vi "1D数组排序[U32].vi"(8 "error in (no error)":errorcluster caption="错误输入（无错误）", 9 "升降序":enum16{"升序", "降序"}(ring), 11 "输入数组":u32[](array[numeric])) -> (0 "error out":errorcluster caption="错误输出", 2 "排序后索引":i32[](array[numeric]), 3 "排序后数组":u32[](array[numeric]))   [LabVIEW 2020]
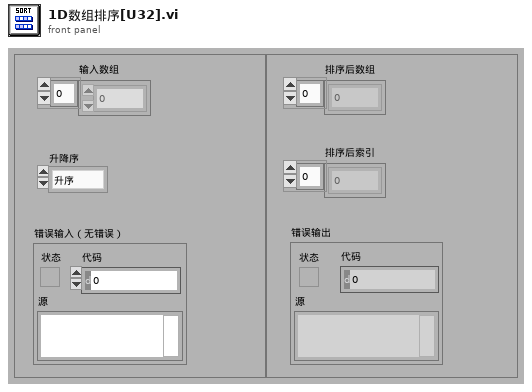
[diagram p1: front panel]
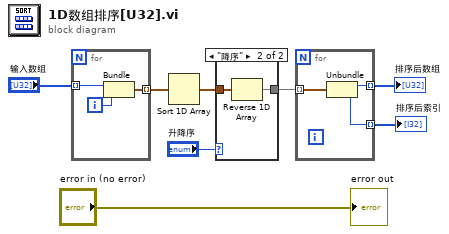
[diagram p0: block diagram]
diagram:
  n1 = for {
    tunnel: "输入数组" -> [w11] mode=indexing
    tunnel: [w9] -> w5 mode=indexing
    i -> [w10]
    n2 = Bundle("数值"=w11, w10) -> (w9:cluster{"数值":u32, i32})  [unwired: 1 in]
  }
  n3 = Sort 1D Array(array=w5) -> (sorted array=w1:cluster{"数值":u32, i32}[])
  n4 = case shown="\"降序\"" "升降序" {
    tunnel: w1 -> [w12 w14]
    tunnel: [w12 w13] -> w2
    frame "升序", Default {
    }
    frame "降序" {
      n5 = Reverse 1D Array(array=w14) -> (reversed array=w13:cluster{"数值":u32, i32}[])
    }
  }
  n6 = for {
    tunnel: w2 -> [w17] mode=indexing
    tunnel: [w16] -> w4 mode=indexing
    tunnel: [w15] -> w3 mode=indexing
    n7 = Unbundle(w17) -> ("数值"=w16:u32, w15:i32)
  }
  "排序后数组" <- w4
  "排序后索引" <- w3
  "error out" <- "error in (no error)"
